vi "colorir_retângulo.vi"(6 "image data":T1, 8 "m (colunas)":i32, 9 "n (linhas)":i32, 10 "Matriz de probabilidades":dbl[][](array[numeric])) -> (3 "data out":u32[][](array[numeric]))   [LabVIEW 2017]
uses:
  <vilib>/picture/picture.llb/imagedata.ctl
  <vilib>/picture/picture.llb/Draw True-Color Pixmap.vi
panel:
  out "campo colorido":picture
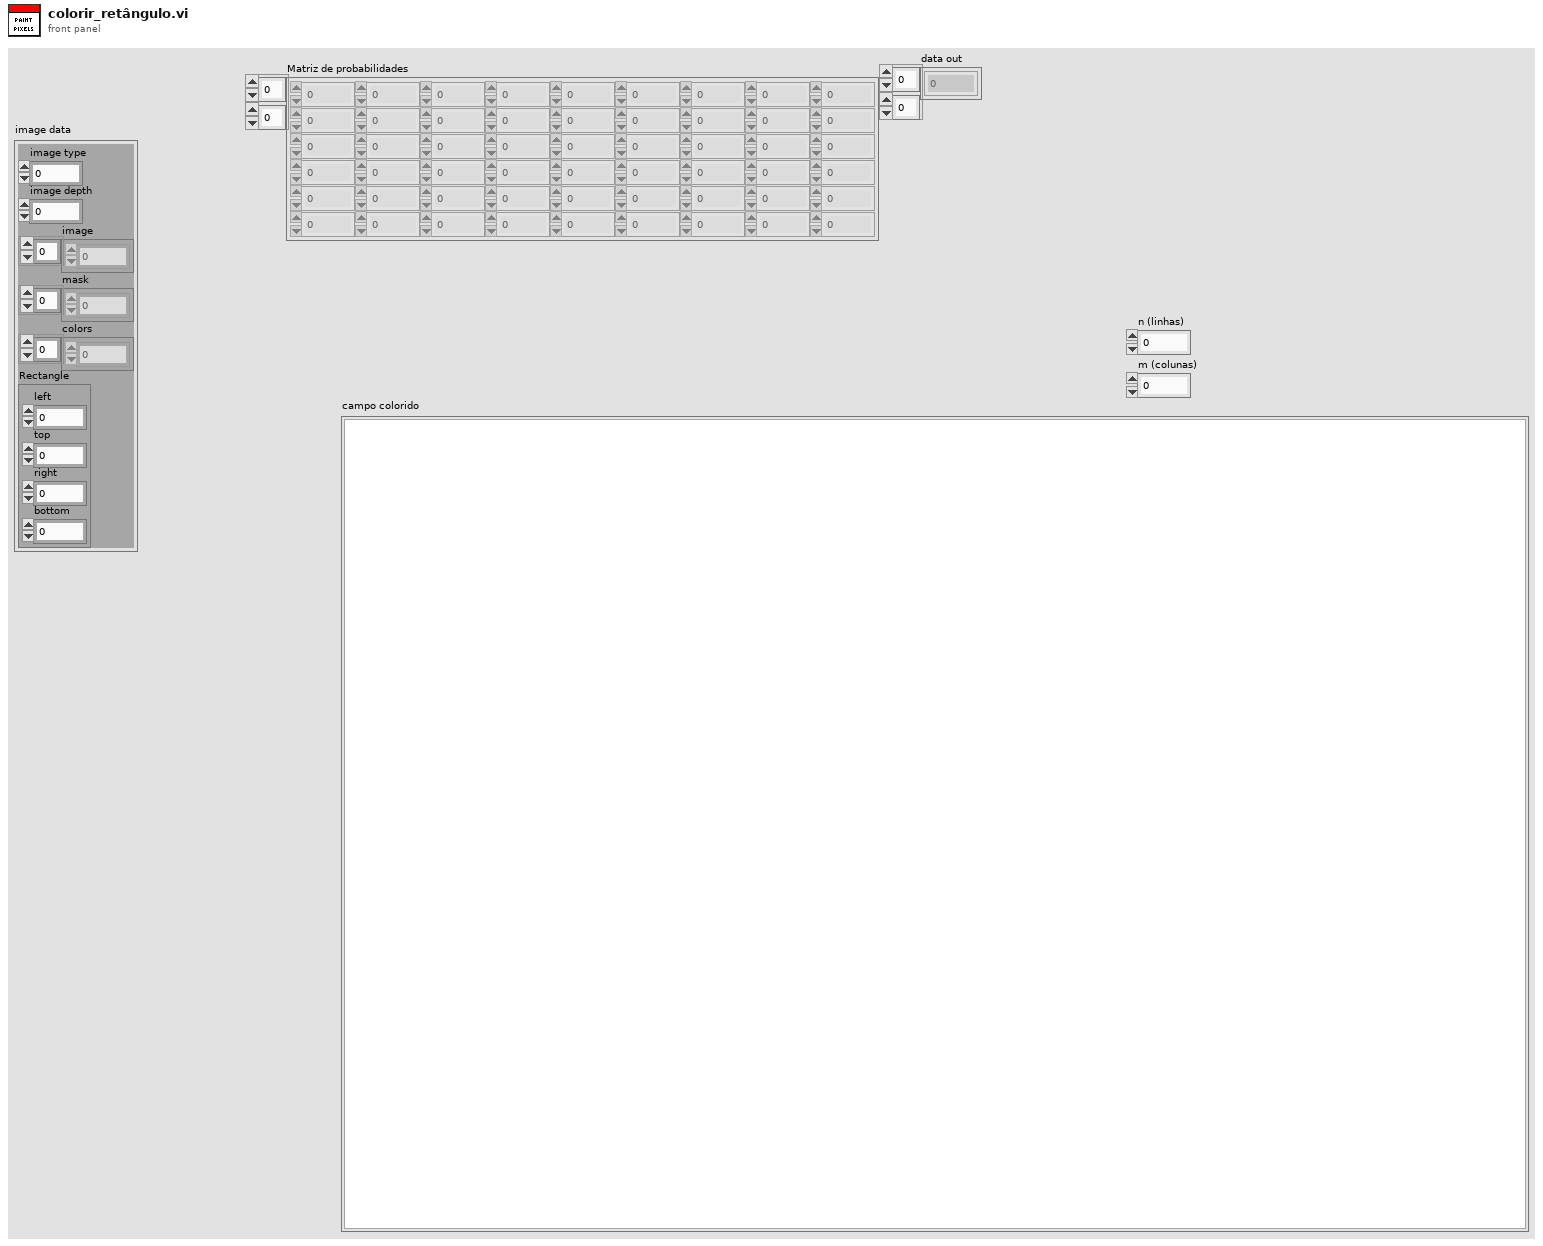
[diagram p1: front panel]
types:
  T1 = typedef "imagedata.ctl" = cluster{"image type":i32, "image depth":i32, "image":u8[], "mask":u8[], "colors":u32[], "Rectangle":cluster{"left":i16, "top":i16, "right":i16, "bottom":i16}}
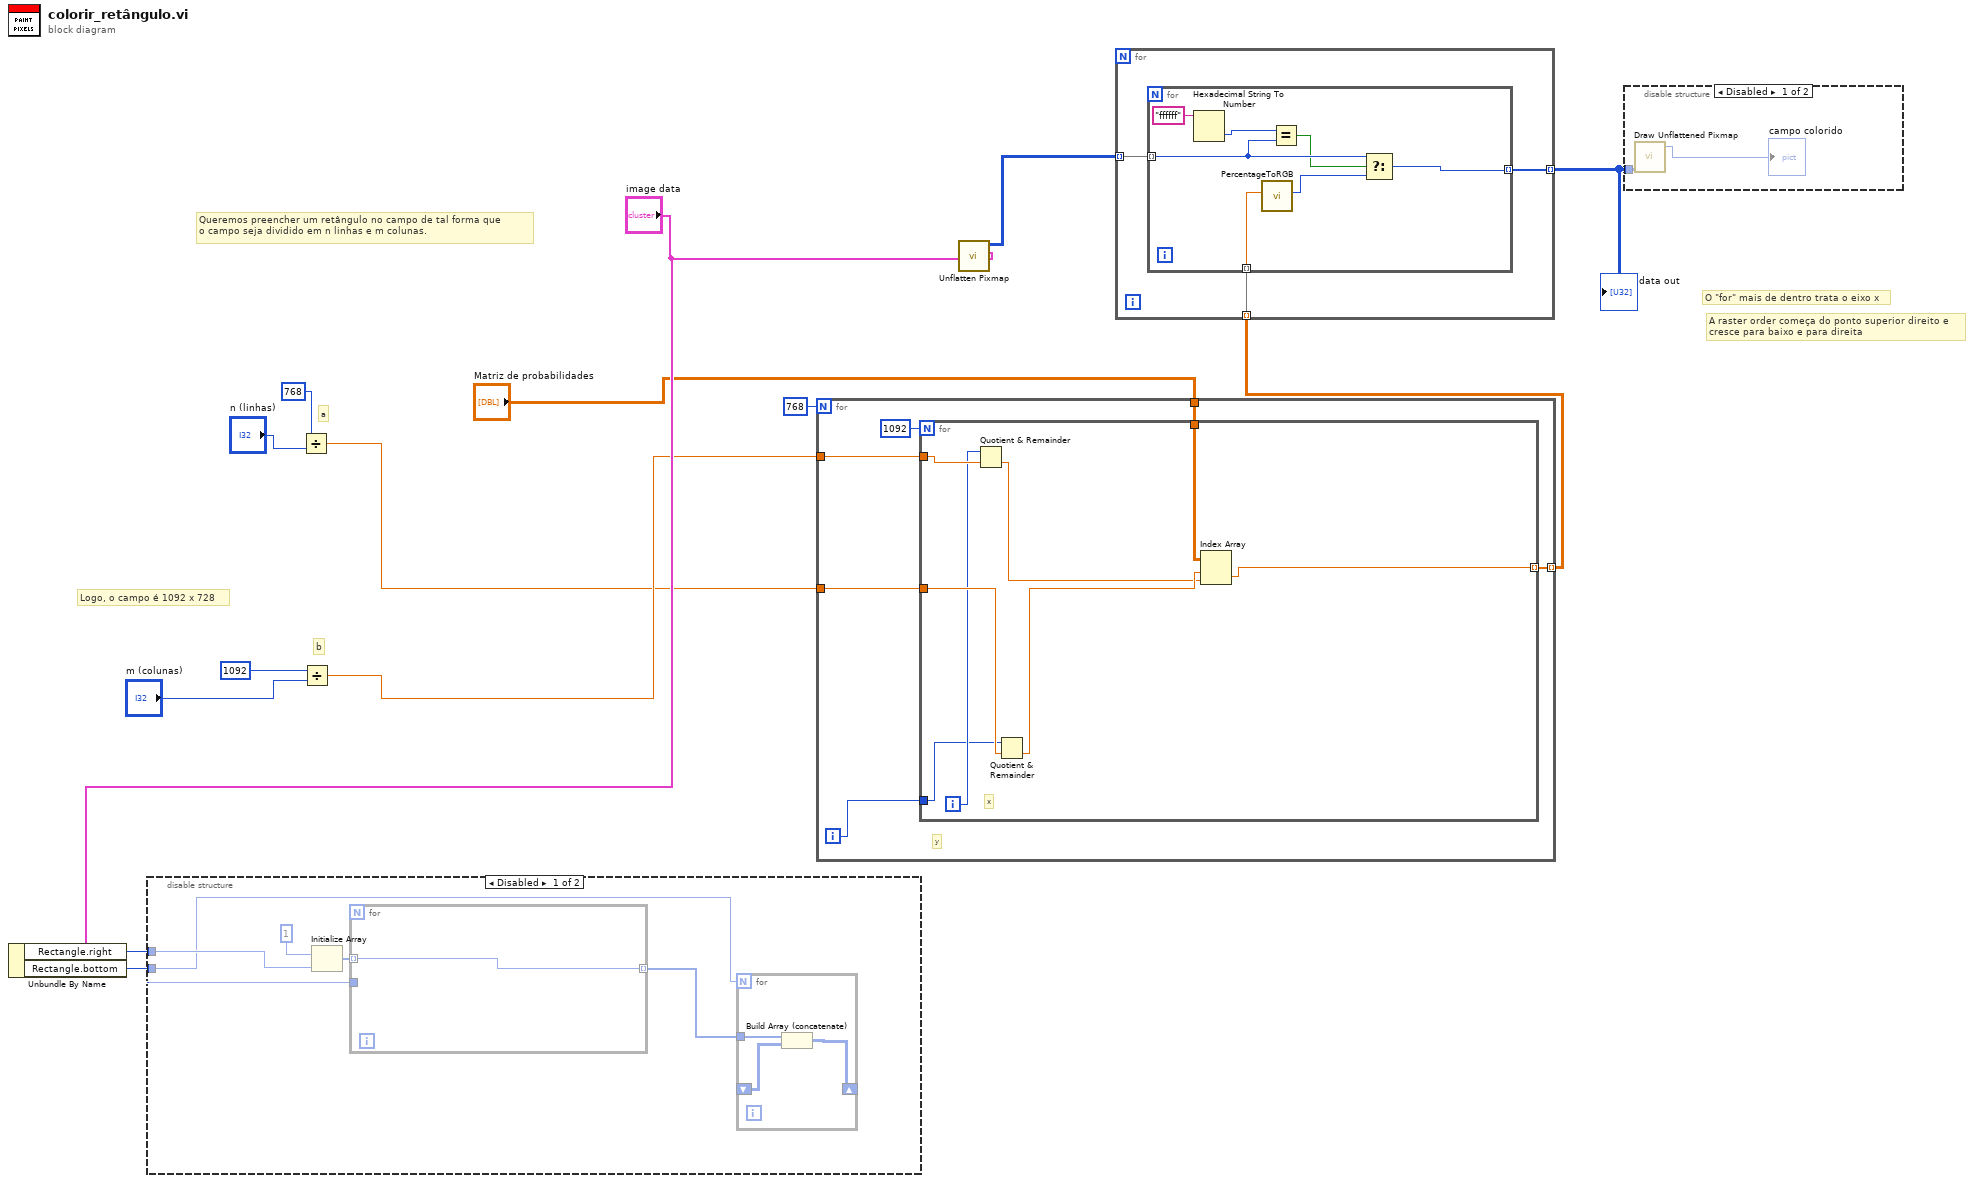
[diagram p0: block diagram]
diagram:
  # "Logo, o campo é 1092 x 728"
  # "b"
  # "a"
  # "Queremos preencher um retângulo no campo de tal forma que\no campo seja dividido em n linhas e m colunas."
  # "A raster order começa do ponto superior direito e\ncresce para baixo e para direita"
  # "O \"for\" mais de dentro trata o eixo x"
  n1 = Unbundle By Name("image data") -> ("Rectangle.right"=w13:i16, "Rectangle.bottom"=w12:i16)
  n2 = disable-structure shown="Disabled" {
    disable-tunnel: w13 -> [w16 _]
    disable-tunnel: w12 -> [w15 _]
    frame Disabled {
      n3 = Initialize Array(1, w16) -> (w19:i32[])
      n4 = for {
        tunnel: w19 -> [w23] mode=indexing
        tunnel: [w23] -> w17 mode=indexing
        tunnel: w16 -> [_]
      }
      n5 = for {
        N: w15 -> [_]
        tunnel: w17 -> [w22]
        shift-right: [w21] -> _
        shift-left: _ -> [w20]
        n6 = Build Array (concatenate)(w22, w20) -> (w21:i32[][])
      }
    }
    frame Enabled {
    }
  }
  n7 = Divide(x=768, y="n (linhas)") -> (x/y=w2:dbl)
  n8 = Divide(x=1092, y="m (colunas)") -> (x/y=w4:dbl)
  n9 = for {
    N: 768 -> [_]
    tunnel: w2 -> [w28]
    tunnel: w4 -> [w27]
    tunnel: "Matriz de probabilidades" -> [w26]
    tunnel: [w25] -> w7 mode=indexing
    i -> [w29]
    # "y"
    n10 = for {
      N: 1092 -> [_]
      tunnel: w29 -> [w33]
      tunnel: w28 -> [w36]
      tunnel: w27 -> [w37]
      tunnel: w26 -> [w35]
      tunnel: [w32] -> w25 mode=indexing
      i -> [w34]
      # "x"
      n11 = Quotient & Remainder(x=w34, y=w37) -> (floor(x/y)=w30:dbl)  [unwired: 1 out]
      n12 = Quotient & Remainder(x=w33, y=w36) -> (floor(x/y)=w31:dbl)  [unwired: 1 out]
      n13 = Index Array(array=w35, index (row)=w31, index (col)=w30) -> (element=w32:dbl)
    }
  }
  n14 = call <vilib>:"Unflatten Pixmap.vi"("image data"="image data") -> ("24-bit pixmap"=w14:u32[][])  [unwired: 4 in, 6 out]
  n15 = for {
    tunnel: w14 -> [w40] mode=indexing
    tunnel: [w39] -> w6 mode=indexing
    tunnel: w7 -> [w38] mode=indexing
    n16 = for {
      tunnel: w40 -> [w45] mode=indexing
      tunnel: [w46] -> w39 mode=indexing
      tunnel: w38 -> [w41] mode=indexing
      n17 = Hexadecimal String To Number(string="ffffff") -> (number=w42:u32)  [unwired: 2 in, 1 out]
      n18 = call "PercentageToRGB.vi"("percentage"=w41) -> ("rgb"=w47:u32)  [unwired: 10 in]
      n19 = Equal?(x=w42, y=w45) -> (x = y?=w44:bool)
      n20 = Select(t=w45, s=w44, f=w47) -> (s? t:f=w46:u32)
    }
  }
  "data out" <- w6
  n21 = disable-structure shown="Disabled" {
    disable-tunnel: w6 -> [w49 _]
    frame Disabled {
      n22 = call-poly <vilib>:"Draw Unflattened Pixmap.vi"("data (RGB format)"=w49) -> ("new picture"=→"campo colorido":picture)  [unwired: 8 in]
    }
    frame Enabled {
    }
  }
